vi "LCDinstall.vi"(8 "error in (no error)":errorcluster, 10 "unsigned byte array":u8[](array[numeric]), 11 "unsigned byte array 2":u8[](array[numeric])) -> (0 "error out":errorcluster)   [LabVIEW 2019]
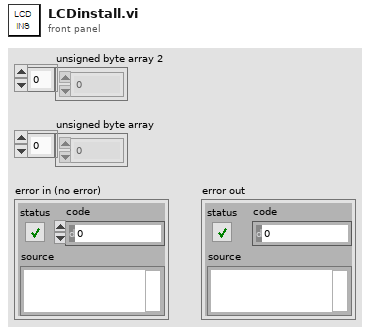
[diagram p1: front panel]
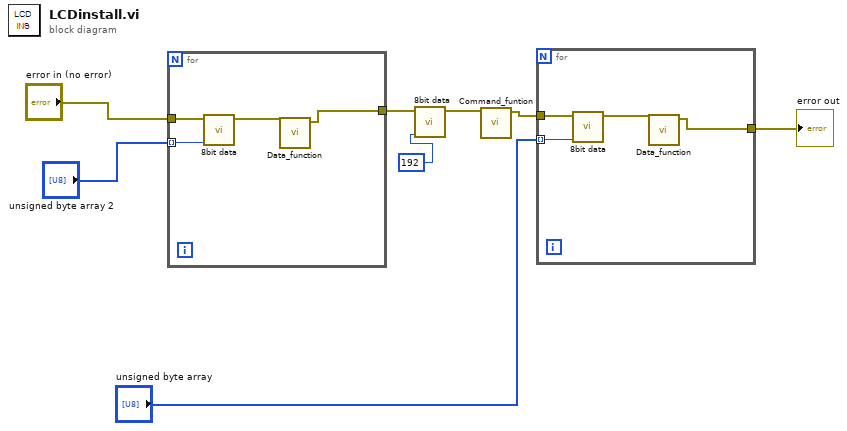
[diagram p0: block diagram]
diagram:
  n1 = for {
    tunnel: "error in (no error)" -> [w12]
    tunnel: [w10] -> w2
    tunnel: "unsigned byte array 2" -> [w9] mode=indexing
    n2 = call "8bit data.vi"("Numeric"=w9, "Error In"=w12) -> ("Error Out"=w11:errorcluster)  [unwired: 9 in]
    n3 = call "Data_function.vi"("Error In"=w11) -> ("Error Out"=w10:errorcluster)  [unwired: 10 in]
  }
  n4 = call "8bit data.vi"("Numeric"=u8 192, "Error In"=w2) -> ("Error Out"=w3:errorcluster)  [unwired: 9 in]
  n5 = call "Command_funtion.vi"("Error In"=w3) -> ("Error Out"=w7:errorcluster)  [unwired: 10 in]
  n6 = for {
    tunnel: "unsigned byte array" -> [w16] mode=indexing
    tunnel: w7 -> [w15]
    tunnel: [w13] -> w8
    n7 = call "8bit data.vi"("Numeric"=w16, "Error In"=w15) -> ("Error Out"=w14:errorcluster)  [unwired: 9 in]
    n8 = call "Data_function.vi"("Error In"=w14) -> ("Error Out"=w13:errorcluster)  [unwired: 10 in]
  }
  "error out" <- w8
